vi "Circle_Wizard.vi"(6 "Coordinates in":dbl[][](array[numeric]), 7 "Device References":refnum<vi>[](array[refnum]), 8 "Device properties":cluster{"Number of axes":i32}[](array[cluster]), 9 "Device parameters":variant[](array[variant]), 10 "Device order":i32[](array[numeric])=[0, 1], 11 "Device description":string[][](array[string])) -> (3 "Coordinates out":dbl[][](array[numeric]))   [LabVIEW 2015]
panel:
  in  "9":bool
  in  "8":bool
  in  "7":bool
  in  "6":bool
  in  "5":bool
  in  "4":bool
  in  "3":bool
  in  "2":bool
  in  "1":bool
  in  "Load parameter":bool
  in  "Cancel Button":bool
  in  "OK Button":bool
  in  "Parameter values":dbl[](array[numeric])=[0.0, 0.0, 0.0, 0.0, 0.0, 0.0, 0.0, 0.0, 0.0]
  out "Parameter names":string[](array[string])
  in  "Scan Pattern":T1(radio)
  # "Parameter names"
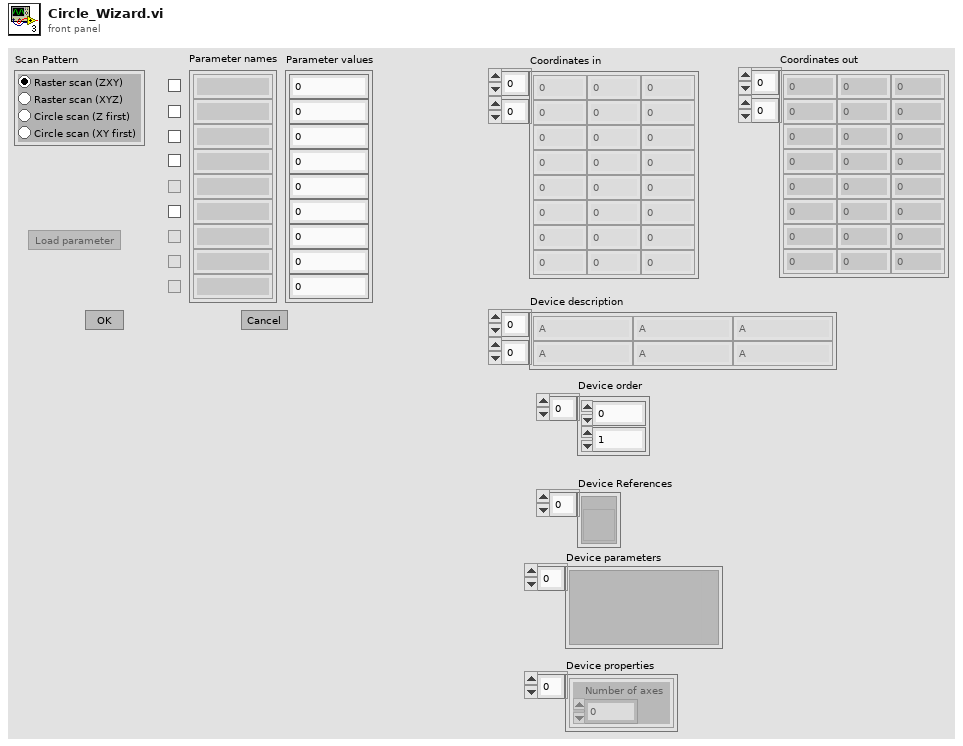
[diagram p1: front panel]
types:
  T1 = enum32{"Raster scan (ZXY)", "Raster scan (XYZ)", "Circle scan (Z first)", "Circle scan (XY first)"}
  T2 = enum8{"Enabled", "Disabled", "Disabled and Grayed Out"}
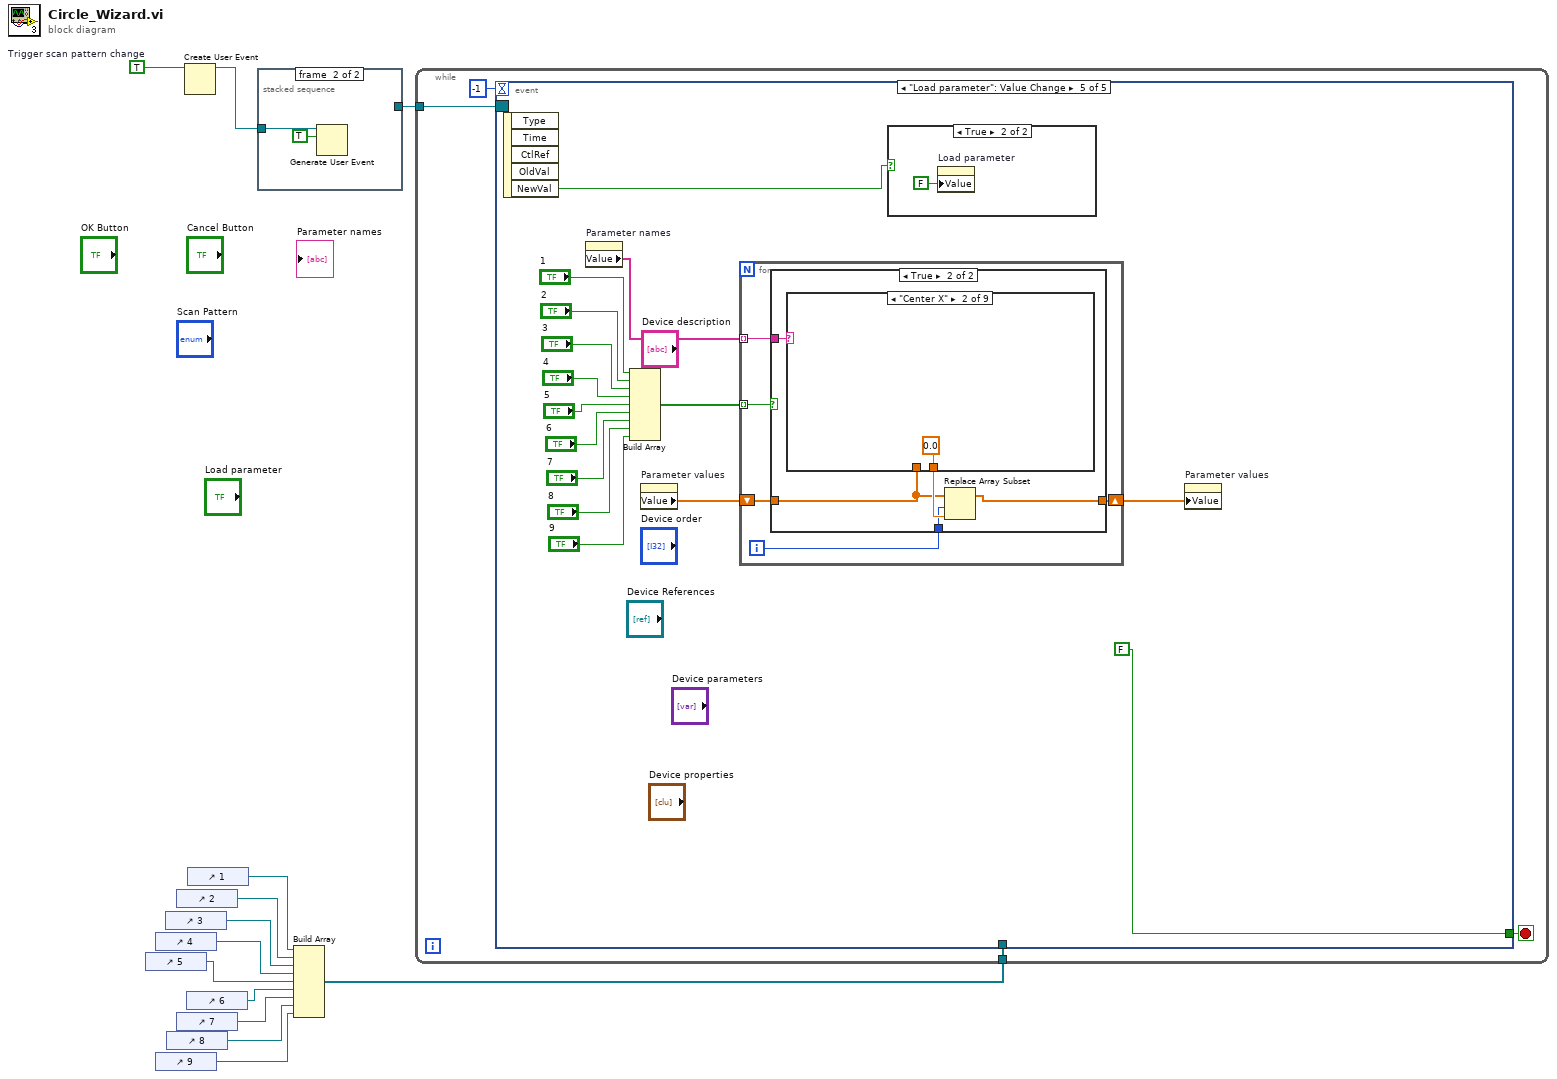
[diagram p0: block diagram]
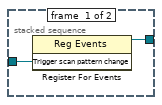
[diagram p2: hidden frame]
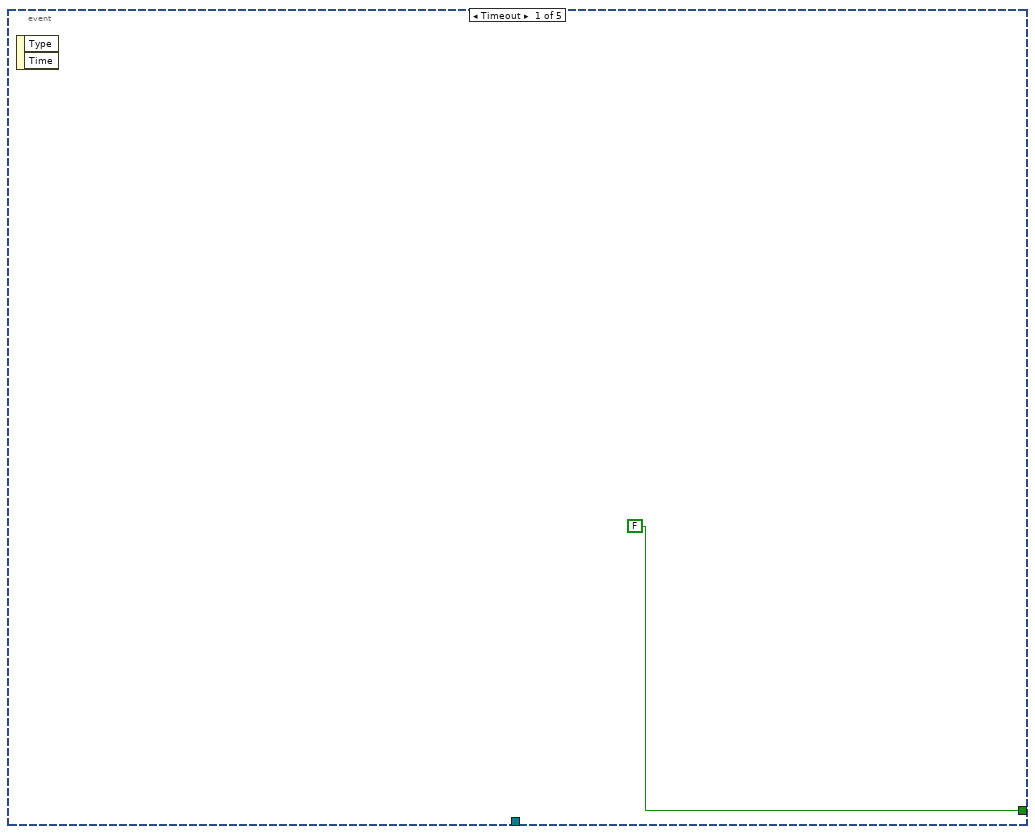
[diagram p3: hidden frame]
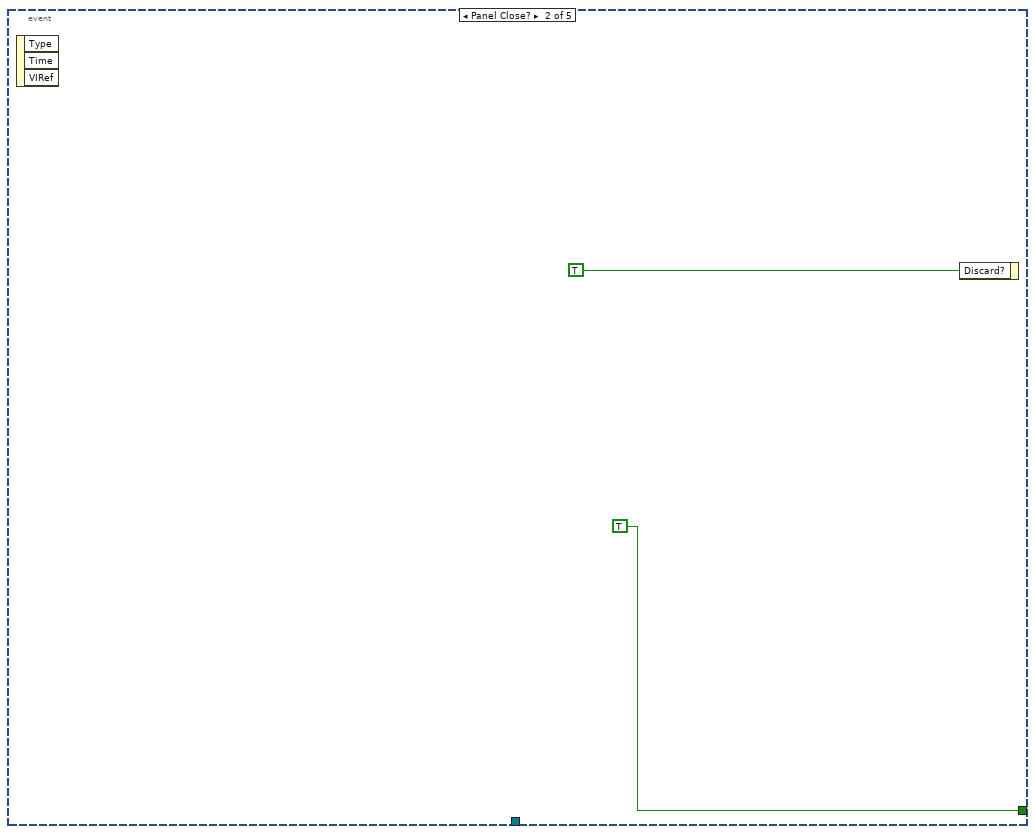
[diagram p4: hidden frame]
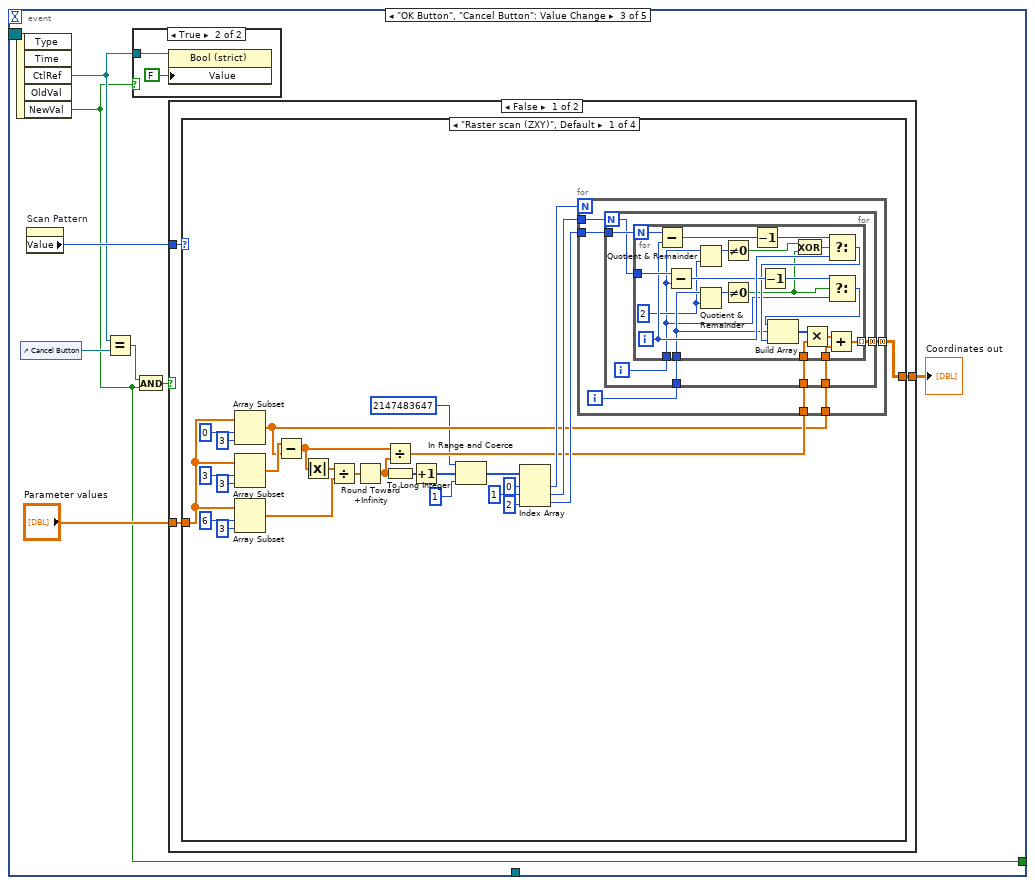
[diagram p5: hidden frame]
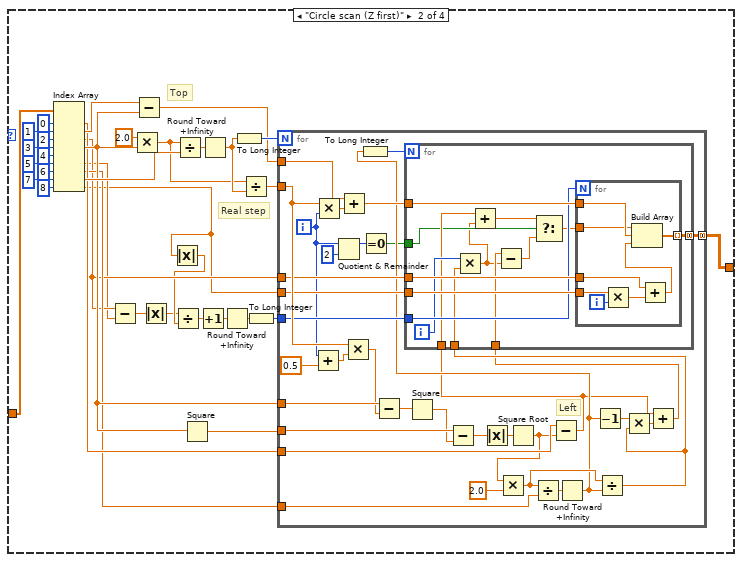
[diagram p7: hidden frame]
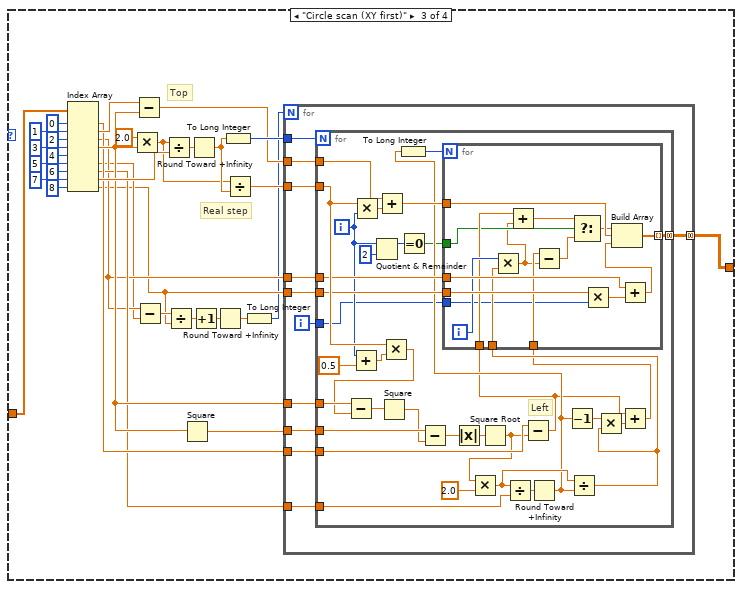
[diagram p8: hidden frame]
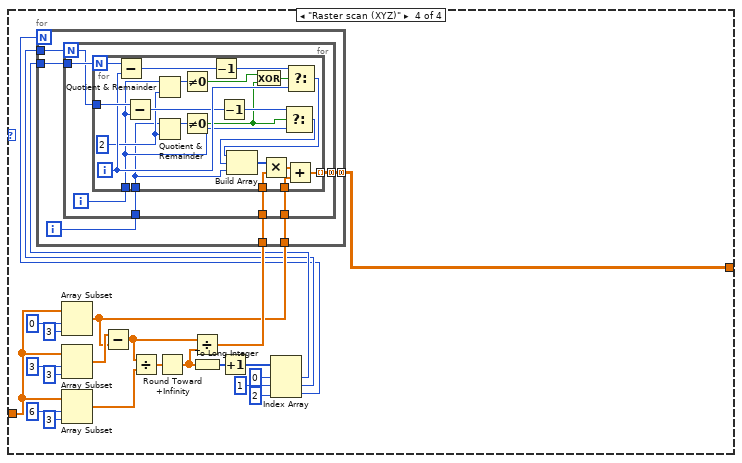
[diagram p9: hidden frame]
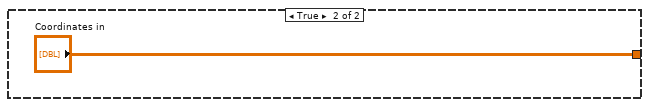
[diagram p10: hidden frame]
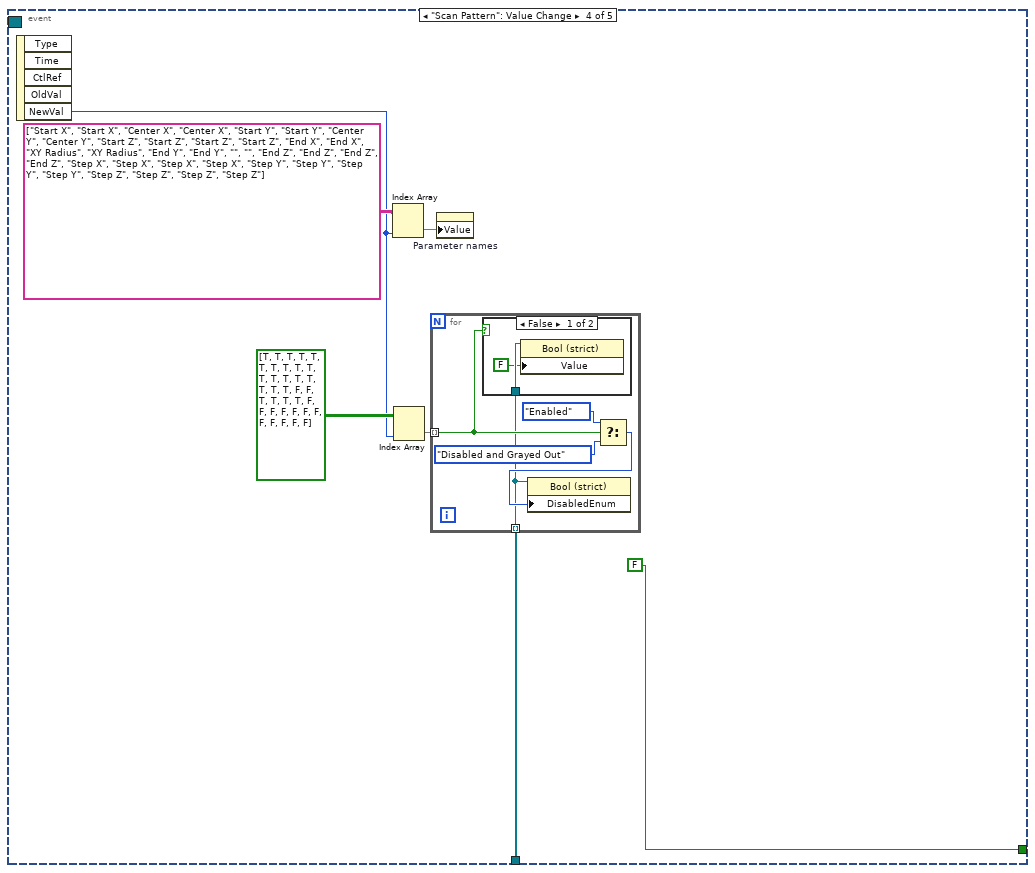
[diagram p11: hidden frame]
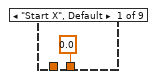
[diagram p15: hidden frame]
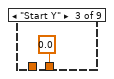
[diagram p16: hidden frame]
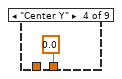
[diagram p17: hidden frame]
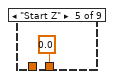
[diagram p18: hidden frame]
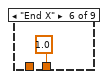
[diagram p19: hidden frame]
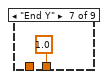
[diagram p20: hidden frame]
diagram:
  w3 = TRUE  # Trigger scan pattern change
  n1 = control-ref of="5"() -> (w9:refnum<vi>)
  n2 = control-ref of="4"() -> (w8:refnum<vi>)
  n3 = control-ref of="9"() -> (w11:refnum<vi>)
  n4 = control-ref of="3"() -> (w7:refnum<vi>)
  n5 = control-ref of="8"() -> (w12:refnum<vi>)
  n6 = control-ref of="2"() -> (w6:refnum<vi>)
  n7 = control-ref of="7"() -> (w13:refnum<vi>)
  n8 = Create User Event(user event datatype=w3) -> (user event=w2:refnum<user-event>)  [unwired: 1 in, 1 out]
  n9 = control-ref of="6"() -> (w10:refnum<vi>)
  n10 = control-ref of="1"() -> (w5:refnum<vi>)
  n11 = stacked-sequence {
    tunnel: w2 -> [w15 w17]
    tunnel: [w14 _] -> w1
    frame #0 {
      n12 = register-events(w15) -> (reference out=w14:refnum<event-registration>)  [unwired: 2 in, 1 out]
    }
    frame #1 {
      n13 = Generate User Event(user event=w17, event data cluster=TRUE ("event data")) -> ()  [unwired: 2 in, 2 out]
    }
  }
  n14 = Build Array(w5, w6, w7, w8, w9, w10, w13, w12, w11) -> (w4:refnum<vi>[])
  n15 = while {
    tunnel: w4 -> [w19]
    tunnel: w1 -> [w18]
    stop <- w21 stop-if-true
    n16 = event shown="[4] \"Load parameter\": Value Change" {
      selector: w18 -> [_ _ _ _ _]
      dyn-events: _ -> [_ _ _ _ _]
      timeout: -1 -> [_ _ _ _ _]
      tunnel: [FALSE TRUE w25 FALSE ("NewVal") FALSE ("NewVal")] -> w21
      tunnel: w19 -> [_ _ _ w342 _]
      event Timeout {
        n17 = event-data() -> ()  [unwired: 1 in, 2 out]
      }
      event Panel Close? {
        n18 = event-data() -> ()  [unwired: 1 in, 3 out]
        n19 = event-data("Discard?"=TRUE) -> ()  [unwired: 1 in, 1 out]
      }
      event "OK Button", "Cancel Button": Value Change {
        n20 = event-data() -> ("CtlRef"=w27:refnum<vi>, "NewVal"=w25:bool)  [unwired: 1 in, 3 out]
        n21 = control-ref of="Cancel Button"() -> (w32:refnum<vi>)
        n22 = property on="Scan Pattern" class="RadioBtnsControl (strict)"() -> ("Value"=w28:T1)  [unwired: 2 in, 2 out]
        n23 = Equal?(x=w27, y=w32) -> (x = y?=w31:bool)
        n24 = case shown="True" w25 {
          tunnel: w27 -> [_ w34]
          frame False {
          }
          frame True {
            n25 = property class="Bool (strict)"(reference=w34, "Value"=FALSE) -> ()  [unwired: 1 in, 2 out]
          }
        }
        n26 = And(x=w31, y=w25) -> (x .and. y?=w30:bool)
        n27 = case shown="False" w30 {
          tunnel: [w35 "Coordinates in"] -> w29
          tunnel: w28 -> [w37 _]
          tunnel: "Parameter values" -> [w36 _]
          frame False {
            n28 = case shown="\"Raster scan (ZXY)\", Default" w37 {
              tunnel: w36 -> [w58 w133 w221 w299]
              tunnel: [w43 w105 w193 w287] -> w35
              frame "Raster scan (ZXY)", Default {
                n29 = Array Subset(array=w58, index=0, length=3) -> (w44:dbl[])
                n30 = Array Subset(array=w58, index=3, length=3) -> (w57:dbl[])
                n31 = Array Subset(array=w58, index=6, length=3) -> (w56:dbl[])
                n32 = Subtract(x=w57, y=w44) -> (x-y=w47:dbl[])
                n33 = Absolute Value(x=w47) -> (abs(x)=w41:dbl[])
                n34 = Divide(x=w41, y=w56) -> (x/y=w55:dbl[])
                n35 = Round Toward +Infinity(x=w55) -> (ceil(x): smallest int >= x=w46:dbl[])
                n36 = Divide(x=w47, y=w46) -> (x/y=w45:dbl[])
                n37 = To Long Integer(number=w46) -> (32bit integer=w54:i32[])
                n38 = Increment(x=w54) -> (x+1=w42:i32[])
                n39 = In Range and Coerce(upper limit=2147483647 ("element"), x=w42, lower limit=1 ("element")) -> (coerced(x)=w40:i32[])  [unwired: 1 out]
                n40 = Index Array(array=w40, index #1=0 ("index"), index #2=1 ("index"), index #3=2 ("index")) -> (element #1=w48:i32, element #2=w49:i32, element #3=w50:i32)
                n41 = for {
                  N: w48 -> [_]
                  tunnel: w50 -> [w70]
                  tunnel: w49 -> [w69]
                  tunnel: w45 -> [w68]
                  tunnel: w44 -> [w67]
                  tunnel: [w66] -> w43 mode=concatenating
                  i -> [w65]
                  n42 = for {
                    N: w69 -> [w71]
                    tunnel: w70 -> [w77]
                    tunnel: w68 -> [w76]
                    tunnel: w67 -> [w75]
                    tunnel: [w74] -> w66 mode=concatenating
                    tunnel: w65 -> [w72]
                    i -> [w73]
                    n43 = for {
                      N: w77 -> [w94]
                      tunnel: w76 -> [w98]
                      tunnel: w75 -> [w96]
                      tunnel: [w95] -> w74 mode=indexing
                      tunnel: w73 -> [w85]
                      tunnel: w72 -> [w87]
                      tunnel: w71 -> [w93]
                      i -> [w92]
                      w86 = 2 ("y")
                      n44 = Subtract(x=w94, y=w92) -> (x-y=w88:i32)
                      n45 = Subtract(x=w93, y=w85) -> (x-y=w91:i32)
                      n46 = Quotient & Remainder(x=w85, y=w86) -> (x-y*floor(x/y)=w83:i32)  [unwired: 1 out]
                      n47 = Quotient & Remainder(x=w87, y=w86) -> (x-y*floor(x/y)=w84:i32)  [unwired: 1 out]
                      n48 = Not Equal To 0?(x=w83) -> (x != 0?=w79:bool)
                      n49 = Not Equal To 0?(x=w84) -> (x != 0?=w78:bool)
                      n50 = Decrement(x=w88) -> (x-1=w82:i32)
                      n51 = Decrement(x=w91) -> (x-1=w81:i32)
                      n52 = Exclusive Or(1:w78, 2:w79) -> (0:w80:bool)
                      n53 = Select(t=w82, s=w80, f=w92) -> (s? t:f=w89:i32)
                      n54 = Select(t=w81, s=w78, f=w85) -> (s? t:f=w90:i32)
                      n55 = Build Array(w90, w87, w89) -> (w99:i32[])
                      n56 = Multiply(x=w99, y=w98) -> (x*y=w97:dbl[])
                      n57 = Add(x=w97, y=w96) -> (x+y=w95:dbl[])
                    }
                  }
                }
              }
              frame "Circle scan (Z first)" {
                # "Real step"
                # "Top"
                n58 = Index Array(array=w133, index #1=0 ("index"), index #2=1 ("index"), index #3=2 ("index"), index #4=3 ("index"), index #5=4 ("index"), index #6=5 ("index"), index #7=6 ("index"), index #8=7 ("index"), index #9=8 ("index")) -> (element #1=w113:dbl, element #2=w118:dbl, element #3=w111:dbl, element #4=w114:dbl, element #6=w110:dbl, element #7=w112:dbl, element #8=w120:dbl, element #9=w102:dbl)  [unwired: 1 out]
                n59 = Subtract(x=w111, y=w110) -> (x-y=w109:dbl)
                n60 = Multiply(x=2.0, y=w114) -> (x*y=w103:dbl)
                n61 = Subtract(x=w118, y=w114) -> (x-y=w117:dbl)
                n62 = Absolute Value(x=w109) -> (abs(x)=w100:dbl)
                n63 = Absolute Value(x=w102) -> (abs(x)=w101:dbl)
                n64 = Divide(x=w100, y=w101) -> (x/y=w108:dbl)
                n65 = Divide(x=w103, y=w120) -> (x/y=w122:dbl)
                n66 = Square(x=w114) -> (x^2=w115:dbl)
                n67 = Increment(x=w108) -> (x+1=w104:dbl)
                n68 = Round Toward +Infinity(x=w122) -> (ceil(x): smallest int >= x=w119:dbl)
                n69 = Round Toward +Infinity(x=w104) -> (ceil(x): smallest int >= x=w107:dbl)
                n70 = To Long Integer(number=w119) -> (32bit integer=w121:i32)
                n71 = Divide(x=w103, y=w119) -> (x/y=w116:dbl)
                n72 = To Long Integer(number=w107) -> (32bit integer=w106:i32)
                n73 = for {
                  N: w121 -> [_]
                  tunnel: w117 -> [w166]
                  tunnel: w116 -> [w161]
                  tunnel: w115 -> [w164]
                  tunnel: w114 -> [w160]
                  tunnel: w113 -> [w147]
                  tunnel: w112 -> [w152]
                  tunnel: w102 -> [w150]
                  tunnel: w111 -> [w149]
                  tunnel: w106 -> [w148]
                  tunnel: [w146] -> w105 mode=concatenating
                  i -> [w142]
                  # "Left"
                  n74 = Add(x=w142, y=0.5) -> (x+y=w162:dbl)
                  n75 = Multiply(x=w161, y=w142) -> (x*y=w167:dbl)
                  n76 = Quotient & Remainder(x=w142, y=2) -> (x-y*floor(x/y)=w140:i32)  [unwired: 1 out]
                  n77 = Add(x=w166, y=w167) -> (x+y=w165:dbl)
                  n78 = Multiply(x=w161, y=w162) -> (x*y=w159:dbl)
                  n79 = Equal To 0?(x=w140) -> (x = 0?=w139:bool)
                  n80 = Subtract(x=w160, y=w159) -> (x-y=w158:dbl)
                  n81 = Square(x=w158) -> (x^2=w157:dbl)
                  n82 = Subtract(x=w164, y=w157) -> (x-y=w156:dbl)
                  n83 = Absolute Value(x=w156) -> (abs(x)=w155:dbl)
                  n84 = Square Root(x=w155) -> (sqrt(x)=w137:dbl)
                  n85 = Multiply(x=w137, y=2.0) -> (x*y=w145:dbl)
                  n86 = Divide(x=w145, y=w152) -> (x/y=w153:dbl)
                  n87 = Subtract(x=w147, y=w137) -> (x-y=w135:dbl)
                  n88 = Round Toward +Infinity(x=w153) -> (ceil(x): smallest int >= x=w143:dbl)
                  n89 = To Long Integer(number=w143) -> (32bit integer=w151:i32)
                  n90 = Decrement(x=w143) -> (x-1=w134:dbl)
                  n91 = Divide(x=w145, y=w143) -> (x/y=w144:dbl)
                  n92 = Multiply(x=w134, y=w144) -> (x*y=w138:dbl)
                  n93 = Add(x=w135, y=w138) -> (x+y=w136:dbl)
                  n94 = for {
                    N: w151 -> [_]
                    tunnel: w165 -> [w181]
                    tunnel: w135 -> [w176]
                    tunnel: w150 -> [w180]
                    tunnel: w149 -> [w179]
                    tunnel: w148 -> [w178]
                    tunnel: [w175] -> w146 mode=concatenating
                    tunnel: w144 -> [w174]
                    tunnel: w139 -> [w171]
                    tunnel: w136 -> [w169]
                    i -> [w177]
                    n95 = Multiply(x=w177, y=w174) -> (x*y=w168:dbl)
                    n96 = Add(x=w176, y=w168) -> (x+y=w173:dbl)
                    n97 = Subtract(x=w169, y=w168) -> (x-y=w170:dbl)
                    n98 = Select(t=w173, s=w171, f=w170) -> (s? t:f=w172:dbl)
                    n99 = for {
                      N: w178 -> [_]
                      tunnel: w181 -> [w189]
                      tunnel: w180 -> [w186]
                      tunnel: w179 -> [w185]
                      tunnel: w172 -> [w183]
                      tunnel: [w182] -> w175 mode=indexing
                      i -> [w188]
                      n100 = Multiply(x=w186, y=w188) -> (x*y=w187:dbl)
                      n101 = Add(x=w185, y=w187) -> (x+y=w184:dbl)
                      n102 = Build Array(w183, w189, w184) -> (w182:dbl[])
                    }
                  }
                }
              }
              frame "Circle scan (XY first)" {
                # "Real step"
                # "Top"
                n103 = Index Array(array=w221, index #1=0 ("index"), index #2=1 ("index"), index #3=2 ("index"), index #4=3 ("index"), index #5=4 ("index"), index #6=5 ("index"), index #7=6 ("index"), index #8=7 ("index"), index #9=8 ("index")) -> (element #1=w201:dbl, element #2=w206:dbl, element #3=w199:dbl, element #4=w202:dbl, element #6=w198:dbl, element #7=w200:dbl, element #8=w208:dbl, element #9=w196:dbl)  [unwired: 1 out]
                n104 = Multiply(x=2.0, y=w202) -> (x*y=w191:dbl)
                n105 = Subtract(x=w206, y=w202) -> (x-y=w205:dbl)
                n106 = Subtract(x=w199, y=w198) -> (x-y=w197:dbl)
                n107 = Divide(x=w191, y=w208) -> (x/y=w210:dbl)
                n108 = Divide(x=w197, y=w196) -> (x/y=w195:dbl)
                n109 = Square(x=w202) -> (x^2=w203:dbl)
                n110 = Round Toward +Infinity(x=w210) -> (ceil(x): smallest int >= x=w207:dbl)
                n111 = Increment(x=w195) -> (x+1=w192:dbl)
                n112 = Round Toward +Infinity(x=w192) -> (ceil(x): smallest int >= x=w194:dbl)
                n113 = To Long Integer(number=w207) -> (32bit integer=w209:i32)
                n114 = Divide(x=w191, y=w207) -> (x/y=w204:dbl)
                n115 = To Long Integer(number=w194) -> (32bit integer=w190:i32)
                n116 = for {
                  N: w190 -> [_]
                  tunnel: w209 -> [w232]
                  tunnel: w205 -> [w231]
                  tunnel: w204 -> [w230]
                  tunnel: w203 -> [w229]
                  tunnel: w202 -> [w228]
                  tunnel: w201 -> [w227]
                  tunnel: w200 -> [w226]
                  tunnel: w199 -> [w225]
                  tunnel: w196 -> [w224]
                  tunnel: [w223] -> w193 mode=concatenating
                  i -> [w222]
                  n117 = for {
                    N: w232 -> [_]
                    tunnel: w231 -> [w265]
                    tunnel: w230 -> [w260]
                    tunnel: w229 -> [w263]
                    tunnel: w228 -> [w259]
                    tunnel: w227 -> [w248]
                    tunnel: w226 -> [w252]
                    tunnel: w224 -> [w250]
                    tunnel: w225 -> [w249]
                    tunnel: [w247] -> w223 mode=concatenating
                    tunnel: w222 -> [w233]
                    i -> [w243]
                    # "Left"
                    n118 = Add(x=w243, y=0.5) -> (x+y=w261:dbl)
                    n119 = Multiply(x=w260, y=w243) -> (x*y=w266:dbl)
                    n120 = Quotient & Remainder(x=w243, y=2) -> (x-y*floor(x/y)=w241:i32)  [unwired: 1 out]
                    n121 = Add(x=w265, y=w266) -> (x+y=w264:dbl)
                    n122 = Multiply(x=w260, y=w261) -> (x*y=w234:dbl)
                    n123 = Subtract(x=w259, y=w234) -> (x-y=w258:dbl)
                    n124 = Square(x=w258) -> (x^2=w257:dbl)
                    n125 = Equal To 0?(x=w241) -> (x = 0?=w240:bool)
                    n126 = Subtract(x=w263, y=w257) -> (x-y=w256:dbl)
                    n127 = Absolute Value(x=w256) -> (abs(x)=w255:dbl)
                    n128 = Square Root(x=w255) -> (sqrt(x)=w238:dbl)
                    n129 = Multiply(x=w238, y=2.0) -> (x*y=w246:dbl)
                    n130 = Divide(x=w246, y=w252) -> (x/y=w253:dbl)
                    n131 = Subtract(x=w248, y=w238) -> (x-y=w236:dbl)
                    n132 = Round Toward +Infinity(x=w253) -> (ceil(x): smallest int >= x=w244:dbl)
                    n133 = To Long Integer(number=w244) -> (32bit integer=w251:i32)
                    n134 = Decrement(x=w244) -> (x-1=w235:dbl)
                    n135 = Divide(x=w246, y=w244) -> (x/y=w245:dbl)
                    n136 = Multiply(x=w235, y=w245) -> (x*y=w239:dbl)
                    n137 = Add(x=w236, y=w239) -> (x+y=w237:dbl)
                    n138 = for {
                      N: w251 -> [_]
                      tunnel: w264 -> [w282]
                      tunnel: w236 -> [w278]
                      tunnel: w250 -> [w281]
                      tunnel: w249 -> [w280]
                      tunnel: [w277] -> w247 mode=indexing
                      tunnel: w245 -> [w276]
                      tunnel: w240 -> [w273]
                      tunnel: w237 -> [w271]
                      tunnel: w233 -> [w267]
                      i -> [w279]
                      n139 = Multiply(x=w279, y=w276) -> (x*y=w270:dbl)
                      n140 = Add(x=w278, y=w270) -> (x+y=w275:dbl)
                      n141 = Subtract(x=w271, y=w270) -> (x-y=w272:dbl)
                      n142 = Select(t=w275, s=w273, f=w272) -> (s? t:f=w274:dbl)
                      n143 = Multiply(x=w281, y=w267) -> (x*y=w269:dbl)
                      n144 = Add(x=w280, y=w269) -> (x+y=w268:dbl)
                      n145 = Build Array(w274, w282, w268) -> (w277:dbl[])
                    }
                  }
                }
              }
              frame "Raster scan (XYZ)" {
                n146 = Array Subset(array=w299, index=0, length=3) -> (w288:dbl[])
                n147 = Array Subset(array=w299, index=3, length=3) -> (w298:dbl[])
                n148 = Array Subset(array=w299, index=6, length=3) -> (w297:dbl[])
                n149 = Subtract(x=w298, y=w288) -> (x-y=w291:dbl[])
                n150 = Divide(x=w291, y=w297) -> (x/y=w296:dbl[])
                n151 = Round Toward +Infinity(x=w296) -> (ceil(x): smallest int >= x=w290:dbl[])
                n152 = Divide(x=w291, y=w290) -> (x/y=w289:dbl[])
                n153 = To Long Integer(number=w290) -> (32bit integer=w295:i32[])
                n154 = Increment(x=w295) -> (x+1=w286:i32[])
                n155 = Index Array(array=w286, index #1=0 ("index"), index #2=1 ("index"), index #3=2 ("index")) -> (element #1=w285:i32, element #2=w284:i32, element #3=w283:i32)
                n156 = for {
                  N: w283 -> [_]
                  tunnel: w285 -> [w311]
                  tunnel: w284 -> [w310]
                  tunnel: w289 -> [w309]
                  tunnel: w288 -> [w308]
                  tunnel: [w307] -> w287 mode=concatenating
                  i -> [w306]
                  n157 = for {
                    N: w310 -> [w312]
                    tunnel: w311 -> [w318]
                    tunnel: w309 -> [w317]
                    tunnel: w308 -> [w316]
                    tunnel: [w315] -> w307 mode=concatenating
                    tunnel: w306 -> [w313]
                    i -> [w314]
                    n158 = for {
                      N: w318 -> [w335]
                      tunnel: w317 -> [w339]
                      tunnel: w316 -> [w337]
                      tunnel: [w336] -> w315 mode=indexing
                      tunnel: w314 -> [w329]
                      tunnel: w313 -> [w319]
                      tunnel: w312 -> [w334]
                      i -> [w333]
                      w330 = 2 ("y")
                      n159 = Subtract(x=w335, y=w333) -> (x-y=w331:i32)
                      n160 = Subtract(x=w334, y=w329) -> (x-y=w332:i32)
                      n161 = Quotient & Remainder(x=w329, y=w330) -> (x-y*floor(x/y)=w327:i32)  [unwired: 1 out]
                      n162 = Quotient & Remainder(x=w319, y=w330) -> (x-y*floor(x/y)=w328:i32)  [unwired: 1 out]
                      n163 = Not Equal To 0?(x=w327) -> (x != 0?=w323:bool)
                      n164 = Not Equal To 0?(x=w328) -> (x != 0?=w322:bool)
                      n165 = Decrement(x=w331) -> (x-1=w326:i32)
                      n166 = Decrement(x=w332) -> (x-1=w325:i32)
                      n167 = Exclusive Or(1:w322, 2:w323) -> (0:w324:bool)
                      n168 = Select(t=w325, s=w322, f=w329) -> (s? t:f=w320:i32)
                      n169 = Select(t=w326, s=w324, f=w333) -> (s? t:f=w321:i32)
                      n170 = Build Array(w321, w320, w319) -> (w340:i32[])
                      n171 = Multiply(x=w340, y=w339) -> (x*y=w338:dbl[])
                      n172 = Add(x=w338, y=w337) -> (x+y=w336:dbl[])
                    }
                  }
                }
              }
            }
          }
          frame True {
          }
        }
        "Coordinates out" <- w29
      }
      event "Scan Pattern": Value Change {
        n173 = event-data() -> ("NewVal"=w344:T1)  [unwired: 1 in, 4 out]
        n174 = Index Array(array=string[][] [["Start X", "Start X", "Center X", "Center X"], ["Start Y", "Start Y", "Center Y", "Center Y"], ["Start Z", "Start Z", "Start Z", "Start Z"], ["End X", "End X", "XY Radius", "XY Radius"], ["End Y", "End Y", "", ""], ["End Z", "End Z", "End Z", "End Z"], ["Step X", "Step X", "Step X", "Step X"], ["Step Y", "Step Y", "Step Y", "Step Y"], ["Step Z", "Step Z", "Step Z", "Step Z"]], index (col)=w344) -> (element=w346:string[])  [unwired: 1 in]
        n175 = Index Array(array=bool[][] [[TRUE, TRUE, TRUE, TRUE], [TRUE, TRUE, TRUE, TRUE], [TRUE, TRUE, TRUE, TRUE], [TRUE, TRUE, TRUE, TRUE], [TRUE, TRUE, FALSE, FALSE], [TRUE, TRUE, TRUE, TRUE], [FALSE, FALSE, FALSE, FALSE], [FALSE, FALSE, FALSE, FALSE], [FALSE, FALSE, FALSE, FALSE]], index (col)=w344) -> (element=w343:bool[])  [unwired: 1 in]
        n176 = for {
          tunnel: w343 -> [w350] mode=indexing
          tunnel: w342 -> [w349] mode=indexing
          n177 = case shown="False" w350 {
            tunnel: w349 -> [w355 _]
            frame False {
              n178 = property class="Bool (strict)"(reference=w355, "Value"=FALSE) -> ()  [unwired: 1 in, 2 out]
            }
            frame True {
            }
          }
          n179 = Select(t=T2."Enabled" ("Disabled"), s=w350, f=T2."Disabled and Grayed Out" ("Disabled")) -> (s? t:f=w351:T2)
          n180 = property class="Bool (strict)"(reference=w349, "DisabledEnum"=w351) -> ()  [unwired: 1 in, 2 out]
        }
        n181 = property on="Parameter names" class="Arr (strict)"("Value"=w346) -> ()  [unwired: 2 in, 2 out]
      }
      event "Load parameter": Value Change {
        n182 = event-data() -> ("NewVal"=w358:bool)  [unwired: 1 in, 4 out]
        n183 = property on="Parameter names" class="Arr (strict)"() -> ("Value"=w360:string[])  [unwired: 2 in, 2 out]
        n184 = Build Array("1", "2", "3", "4", "5", "6", "7", "8", "9") -> (w361:bool[])
        n185 = property on="Parameter values" class="Arr (strict)"() -> ("Value"=w357:dbl[])  [unwired: 2 in, 2 out]
        n186 = for {
          tunnel: w361 -> [w376] mode=indexing
          tunnel: w360 -> [w375] mode=indexing
          shift-right: [w372] -> w356
          shift-left: w357 -> [w373]
          i -> [w374]
          n187 = case shown="True" w376 {
            tunnel: w375 -> [_ w382]
            tunnel: w374 -> [_ w380]
            tunnel: w373 -> [w377 w379]
            tunnel: [w377 w378] -> w372
            frame False {
            }
            frame True {
              n188 = case shown="\"Center X\"" w382 {
                tunnel: [0.0 ("Position out") 0.0 ("Position out") 0.0 ("Position out") 0.0 ("Position out") 0.0 ("Position out") 1.0 ("Position out") 1.0 ("Position out") 1.0 ("Position out") 1.0 ("Position out")] -> w381
                tunnel: w379 -> [_ _ _ _ _ _ _ _ _]
                frame "Start X", Default {
                }
                frame "Center X" {
                }
                frame "Start Y" {
                }
                frame "Center Y" {
                }
                frame "Start Z" {
                }
                frame "End X" {
                }
                frame "End Y" {
                }
                frame "End Z" {
                }
                frame " XY Radius" {
                }
              }
              n189 = Replace Array Subset(array=w379, new element=w381, index=w380) -> (w378:dbl[])
            }
          }
        }
        n190 = case shown="True" w358 {
          frame False {
          }
          frame True {
            n191 = property on="Load parameter" class="Bool (strict)"("Value"=FALSE ("Load parameter")) -> ()  [unwired: 2 in, 2 out]
          }
        }
        n192 = property on="Parameter values" class="Arr (strict)"("Value"=w356) -> ()  [unwired: 2 in, 2 out]
      }
    }
  }
